vi "RunProbeCycle.vi"(10 "UiDefinition":T1) -> ()   [LabVIEW 2020]
uses:
  UIReferences.ctl
  D:/LabviewDXFViewer/LabviewDXFViewer/bin/Release/LabviewDXFViewer.exe
  LabviewDXFViewer/bin/Release/LabviewDXFViewer.exe
  <vilib>/Utility/file.llb/Write Delimited Spreadsheet (string).vi
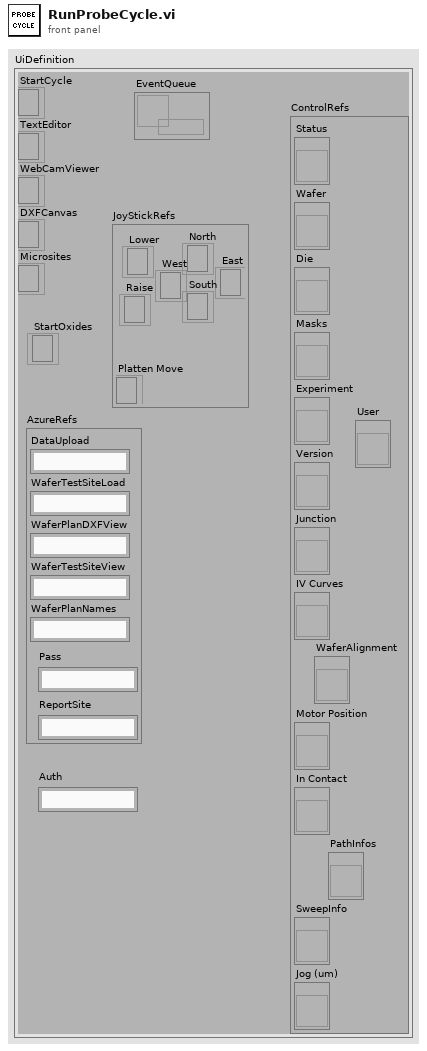
[diagram p1: front panel]
types:
  T1 = typedef "UIReferences.ctl" = cluster{"StartCycle":refnum<k24>, "TextEditor":refnum<k24>, "WebCamViewer":refnum<k24>, "DXFCanvas":refnum<k24>, "Microsites":refnum<k24>, "JoyStickRefs":cluster{"North":refnum<k24>, "Lower":refnum<k24>, "Raise":refnum<k24>, "Platten Move":refnum<k24>, "West":refnum<k24>, "East":refnum<k24>, "South":refnum<k24>}, "AzureRefs":cluster{"DataUpload":string, "WaferTestSiteLoad":string, "WaferPlanDXFView":string, "WaferTestSiteView":string, "WaferPlanNames":string, "Pass":string, "ReportSite":string}, "ControlRefs":cluster{"Status":refnum<vi>, "Wafer":refnum<vi>, "Die":refnum<vi>, "Masks":refnum<vi>, "Experiment":refnum<vi>, "Version":refnum<vi>, "Junction":refnum<vi>, "IV Curves":refnum<vi>, "Motor Position":refnum<vi>, "In Contact":refnum<vi>, "SweepInfo":refnum<vi>, "Jog (um)":refnum<vi>, "PathInfos":refnum<vi>, "User":refnum<vi>, "WaferAlignment":refnum<vi>}, "EventQueue":refnum<queue>, "StartOxides":refnum<k24>, "Auth":string}
  T2 = typedef "WaferAlignmentType.ctl" = cluster{"Wafer Units to microns":dbl, "Rotation Misalign":dbl[], "Scale Misalign":dbl, "Steps Per micron":dbl, "Position 1":i32[], "Position 2":i32[], "Lift Distance":i32, "Position 3":i32[], "Jog Height":i32}
  T3 = cluster{"Current Range":dbl, "Source Measure Unit Channel (0: Channel A)":i32, "Waveform":waveform(dbl), "VISA resource name":refnum<visa-resource-name>, "CodeText":string}
  T4 = cluster{"Die":string, "Wafer":string, "Path":path, "url":string, "Experiment":string, "Version":string, "user":string}
  T5 = cluster{"Coordinates":dbl[], "Junction Name":string, "Orientation":string}[]
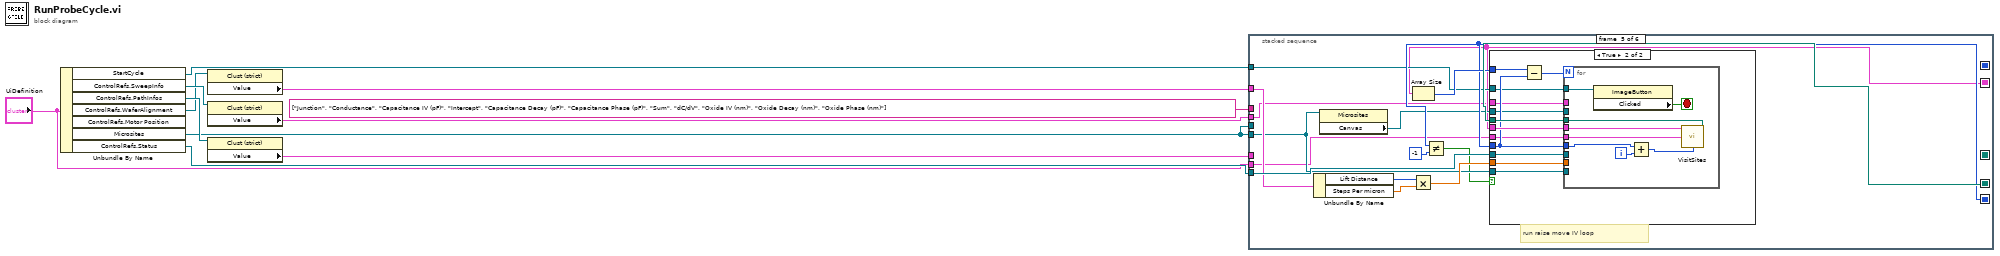
[diagram p0: block diagram]
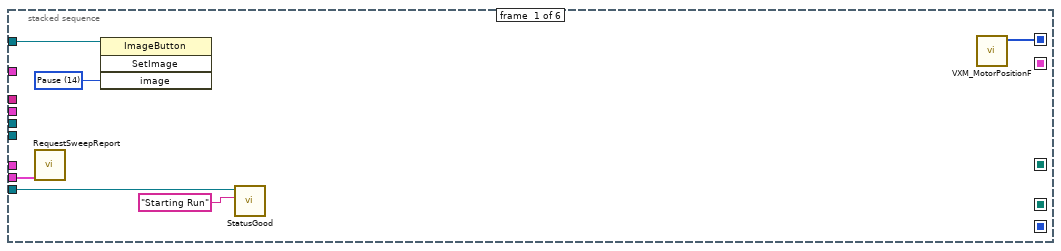
[diagram p2: hidden frame]
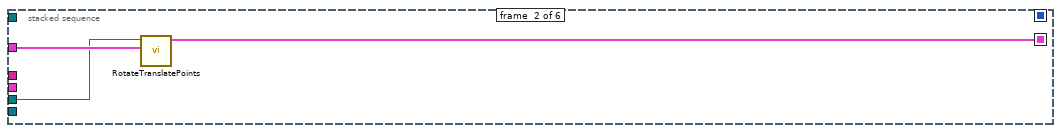
[diagram p3: hidden frame]
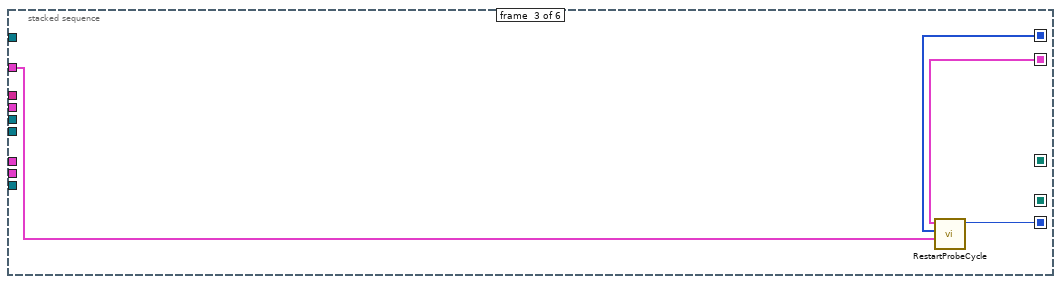
[diagram p4: hidden frame]
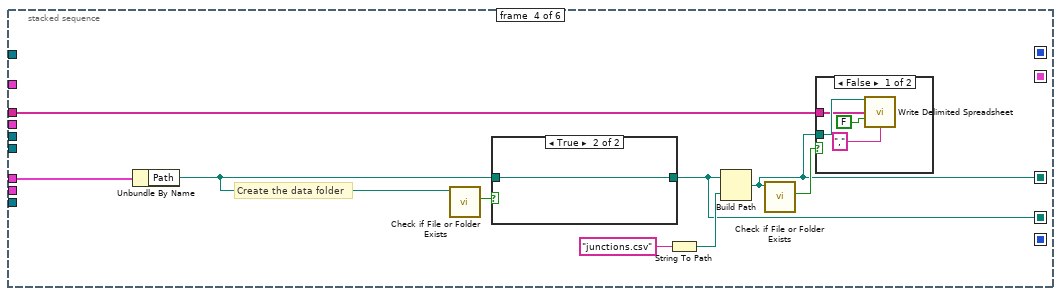
[diagram p5: hidden frame]
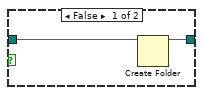
[diagram p7: hidden frame]
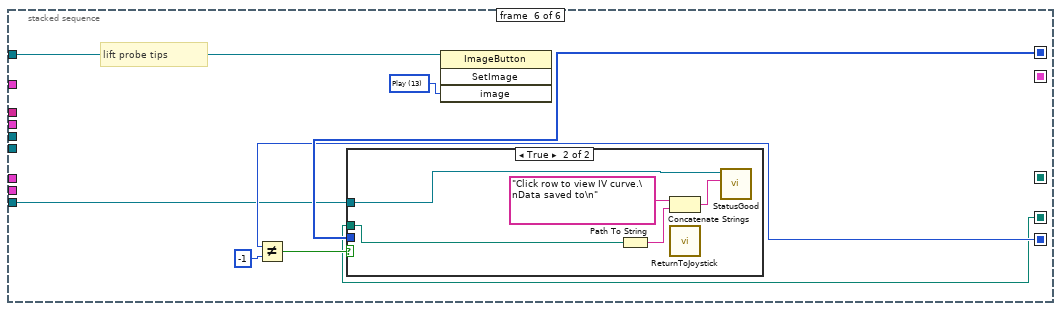
[diagram p9: hidden frame]
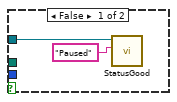
[diagram p10: hidden frame]
diagram:
  n1 = Unbundle By Name("UiDefinition") -> ("StartCycle"=w11:refnum<k24>, "ControlRefs.SweepInfo"=w10:refnum<vi>, "ControlRefs.PathInfos"=w7:refnum<vi>, "ControlRefs.WaferAlignment"=w6:refnum<vi>, "Microsites"=w3:refnum<k24>, "ControlRefs.Status"=w5:refnum<vi>)  [unwired: 1 out]
  n2 = property class="Clust (strict)"(reference=w6) -> ("Value"=w4:T2)  [unwired: 1 in, 2 out]
  n3 = property class="Clust (strict)"(reference=w10) -> ("Value"=w9:T3)  [unwired: 1 in, 2 out]
  n4 = property class="Clust (strict)"(reference=w7) -> ("Value"=w8:T4)  [unwired: 1 in, 2 out]
  n5 = stacked-sequence {
    seq-local: [_ w20 _ _ _ _] -> [_ _ w21 _ w44 _]
    seq-local: [w17 _ _ _ _ _] -> [_ _ w23 _ _ w84]
    seq-local: [_ _ _ w29 _ _] -> [_ _ _ _ w56 w78]
    seq-local: [_ _ w24 _ _ _] -> [_ _ _ _ w54 w82]
    seq-local: [_ _ _ w26 _ _] -> [_ _ _ _ _ _]
    tunnel: w3 -> [_ _ _ _ w45 _]
    tunnel: w8 -> [_ _ _ w30 _ _]
    tunnel: w9 -> [_ _ _ _ w42 _]
    tunnel: w11 -> [w16 _ _ _ w52 w80]
    tunnel: w5 -> [w13 _ _ _ w51 w77]
    tunnel: w4 -> [_ w19 w22 _ w50 _]
    tunnel: w3 -> [_ w18 _ _ _ _]
    tunnel: "UiDefinition" -> [w12 _ _ _ w43 _]
    tunnel: string[] ["Junction", "Conductance", "Capacitance IV (pF)", "Intercept", "Capacitance Decay (pF)", "Capacitance Phase (pF)", "Sum", "dC/dV", "Oxide IV (nm)", "Oxide Decay (nm)", "Oxide Phase (nm)"] -> [_ _ _ w25 _ _]
    frame #0 {
      w15 = 14 items=["Left", "LeftBig", "LeftSmall", "Right", "RightBig", "RightSmall", "Up", "UpBig", "UpSmall", "Down", "DownBig", "DownSmall", "Zero", "Play", "Pause", "Load", "Lower", "Raise", "Home", "Home2"] ("image")
      n6 = call "RequestSweepReport.vi"("UiDefinition 2"=w12) -> ()  [unwired: 11 in]
      n7 = invoke class="ImageButton" method="SetImage"(reference=w16, "image"=w15) -> ()  [unwired: 2 in, 4 out]
      n8 = call "StatusGood.vi"("Text.Text"="Starting Run" ("Run Message"), "String in"=w13) -> ()  [unwired: 10 in]
      n9 = call "VXM_MotorPositionF.vi"() -> ("Position"=w17:i32[])  [unwired: 11 in]
    }
    frame #1 {
      n10 = call "RotateTranslatePoints.vi"("WaferAlignment"=w19, ".NET Refnum in"=w18) -> ("Array"=w20:T5)  [unwired: 9 in]
    }
    frame #2 {
      n11 = call "RestartProbeCycle.vi"("WaferAlignment"=w22, "Position"=w23, "Array"=w21) -> ("Numeric"=w24:i32)  [unwired: 8 in]
    }
    frame #3 {
      # "Create the data folder"
      n12 = Unbundle By Name(w30) -> ("Path"=w28:path)
      n13 = call <vilib>:"Check if File or Folder Exists.vi"("path"=w28) -> ("file or folder exists?"=w33:bool)  [unwired: 8 in, 2 out]
      n14 = case shown="True" w33 {
        tunnel: w28 -> [w39 w40]
        tunnel: [w38 w40] -> w29
        frame False {
          n15 = Create Folder(path (use dialog)=w39) -> (created path=w38:path)  [unwired: 2 in, 2 out]
        }
        frame True {
        }
      }
      n16 = String To Path(string="junctions.csv") -> (path=w32:path)
      n17 = Build Path(base path=w29, name or relative path=w32) -> (appended path=w26:path)
      n18 = call <vilib>:"Check if File or Folder Exists.vi"("path"=w26) -> ("file or folder exists?"=w27:bool)  [unwired: 8 in, 2 out]
      n19 = case shown="False" w27 {
        tunnel: w26 -> [w37 _]
        tunnel: w25 -> [w34 _]
        frame False {
          n20 = call-poly <vilib>:"Write Delimited Spreadsheet.vi"("file path (dialog if empty)"=w37, "1D data"=w34, "append to file? (new file:F)"=FALSE, "delimiter (\\t)"="," ("delimiter (\\t)")) -> ()  [unwired: 10 in, 2 out]
        }
        frame True {
        }
      }
    }
    frame #4 {
      # "run raise move IV loop"
      n21 = Unbundle By Name(w50) -> ("Lift Distance"=w49:i32, "Steps Per micron"=w48:dbl)
      n22 = property class="Microsites"(reference=w45) -> ("Canvas"=w46:refnum<k24>)  [unwired: 1 in, 2 out]
      n23 = Array Size(array=w44) -> (size(s)=w55:i32)
      n24 = Multiply(x=w49, y=w48) -> (x*y=w47:dbl)
      n25 = Not Equal?(x=w54, y=-1) -> (x != y?=w41:bool)
      n26 = case shown="True" w41 {
        tunnel: w44 -> [_ w68]
        tunnel: w45 -> [_ w67]
        tunnel: w56 -> [_ w66]
        tunnel: w54 -> [_ w63]
        tunnel: w55 -> [_ w64]
        tunnel: w42 -> [_ w62]
        tunnel: w52 -> [_ w61]
        tunnel: w51 -> [_ w60]
        tunnel: w47 -> [_ w59]
        tunnel: w46 -> [_ w58]
        tunnel: w43 -> [_ w57]
        frame False {
        }
        frame True {
          n27 = Subtract(x=w64, y=w63) -> (x-y=w65:i32)
          n28 = for {
            N: w65 -> [_]
            tunnel: w59 -> [_]
            tunnel: w68 -> [w73]
            tunnel: w67 -> [_]
            tunnel: w66 -> [w74]
            tunnel: w63 -> [w75]
            tunnel: w62 -> [_]
            tunnel: w61 -> [w71]
            tunnel: w60 -> [_]
            tunnel: w58 -> [_]
            tunnel: w57 -> [w72]
            i -> [w76]
            stop <- w70 stop-if-true
            n29 = property class="ImageButton"(reference=w71) -> ("Clicked"=w70:bool)  [unwired: 1 in, 2 out]
            n30 = Add(x=w75, y=w76) -> (x+y=w69:i32)
            n31 = call "VisitSites.vi"("Microsites"=w73, "Path"=w74, "UiDefinition"=w72, "CurrentPositionIndex"=w69) -> ()  [unwired: 12 in]
          }
        }
      }
    }
    frame #5 {
      w79 = 13 items=["Left", "LeftBig", "LeftSmall", "Right", "RightBig", "RightSmall", "Up", "UpBig", "UpSmall", "Down", "DownBig", "DownSmall", "Zero", "Play", "Pause", "Load", "Lower", "Raise", "Home", "Home2"] ("image")
      # "lift probe tips"
      n32 = Not Equal?(x=w82, y=-1) -> (x != y?=w81:bool)
      n33 = case shown="True" w81 {
        tunnel: w84 -> [_ _]
        tunnel: w78 -> [_ w91]
        tunnel: w77 -> [w86 w90]
        frame False {
          n34 = call "StatusGood.vi"("Text.Text"="Paused", "String in"=w86) -> ()  [unwired: 10 in]
        }
        frame True {
          n35 = Path To String(path=w91) -> (string=w89:string)
          n36 = Concatenate Strings("Click row to view IV curve.\nData saved to\n" ("Text.Text"), w89) -> (w87:string)
          n37 = call "ReturnToJoystick.vi"() -> ()  [unwired: 12 in]
          n38 = call "StatusGood.vi"("Text.Text"=w87, "String in"=w90) -> ()  [unwired: 10 in]
        }
      }
      n39 = invoke class="ImageButton" method="SetImage"(reference=w80, "image"=w79) -> ()  [unwired: 2 in, 4 out]
    }
  }
